vi "BuildMenu3.vi"(8 "Click Type":T1, 9 "Point":T2, 10 "XRef":refnum<vi>, 11 "State In":T10) -> (1 "Show Standard Items? (Popup click only)":bool=TRUE, 2 "Menu Specification":T4)   [LabVIEW 2018, in "Foreign Key Sort.xnode"]
uses:
  Foreign Key Sort.xnode
  State.ctl
  <vilib>/XNodeSupport/XNodeMenuSpecs3.ctl
  <vilib>/XNodeSupport/XNodeMenuSpec3.ctl
  <vilib>/XNodeSupport/XNodeString.ctl
  <vilib>/XNodeSupport/XNodeBool.ctl
  <vilib>/XNodeSupport/XNodeStandardHelpInfo.ctl
  <vilib>/XNodeSupport/XNodePath.ctl
  <vilib>/XNodeSupport/XNodePoint.ctl
  <vilib>/XNodeSupport/XNodeInt.ctl
  <vilib>/XNodeSupport/XNodeClickTypes.ctl
  <vilib>/XNodeSupport/NI_XNodeSupport.lvlib
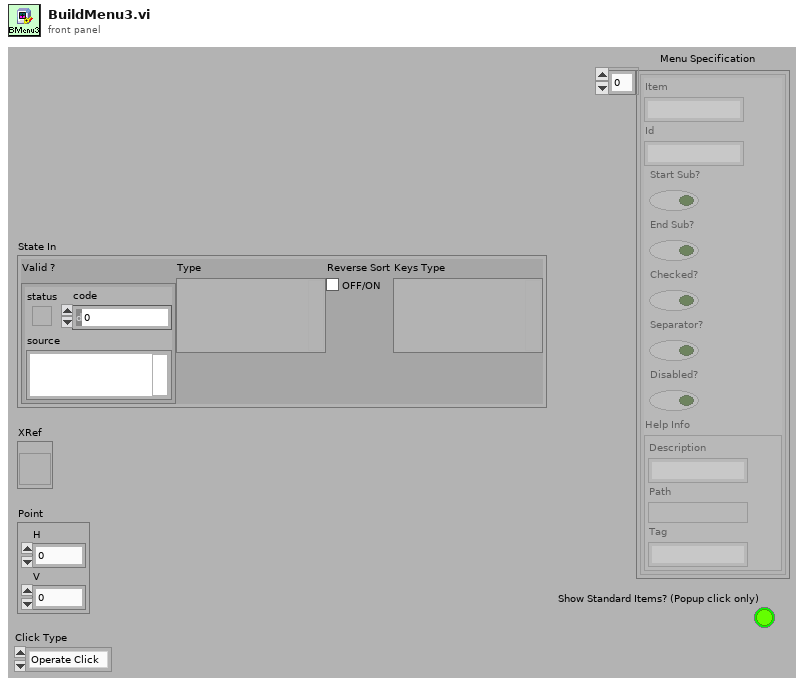
[diagram p1: front panel]
types:
  T1 = typedef "NI_XNodeSupport.lvlib/XNodeClickTypes.ctl" = enum32{"Operate Click", "Popup Click"}
  T2 = typedef "NI_XNodeSupport.lvlib/XNodePoint.ctl" = cluster{"H":T3, "V":T3}
  T3 = typedef "NI_XNodeSupport.lvlib/XNodeInt.ctl" = i32
  T4 = typedef "NI_XNodeSupport.lvlib/XNodeMenuSpecs3.ctl" = T5[]
  T5 = typedef "NI_XNodeSupport.lvlib/XNodeMenuSpec3.ctl" = cluster{"Item":T6, "Id":T6, "Start Sub?":T7, "End Sub?":T7, "Checked?":T7, "Separator?":T7, "Disabled?":T7, "Help Info":T8}
  T6 = typedef "NI_XNodeSupport.lvlib/XNodeString.ctl" = string
  T7 = typedef "NI_XNodeSupport.lvlib/XNodeBool.ctl" = bool
  T8 = typedef "NI_XNodeSupport.lvlib/XNodeStandardHelpInfo.ctl" = cluster{"Description":T6, "Path":T9, "Tag":T6}
  T9 = typedef "NI_XNodeSupport.lvlib/XNodePath.ctl" = path
  T10 = typedef "Foreign Key Sort.xnode/State.ctl" = cluster{"Valid ?":errorcluster, "Type":variant, "Reverse Sort":bool, "Keys Type":variant}
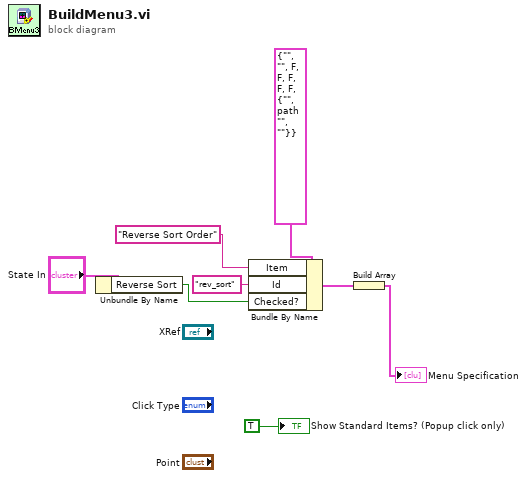
[diagram p0: block diagram]
diagram:
  n1 = Unbundle By Name("State In") -> ("Reverse Sort"=w5:bool)
  n2 = Bundle By Name(cluster=T5 {"Item"="", "Id"="", "Start Sub?"=FALSE, "End Sub?"=FALSE, "Checked?"=FALSE, "Separator?"=FALSE, "Disabled?"=FALSE, "Help Info"={"Description"="", "Path"=path "", "Tag"=""}} ("Menu Item 3"), "Item"=T6 "Reverse Sort Order", "Id"=T6 "rev_sort", "Checked?"=w5) -> (w2:T5)
  n3 = Build Array(w2) -> (→"Menu Specification":T5[])
  "Show Standard Items? (Popup click only)" <- TRUE ("Show Standard Items? (Popup click only)")
